vi "LVClass_CameraSet Get Parameter List.vi"(0 "CameraSet in":refnum<class "CameraSet.lvclass">, 11 "error in (no error)":errorcluster) -> (4 "CameraSet out":refnum<class "CameraSet.lvclass">, 8 "ListOfGettableParameter":T1[](array[typedef]), 15 "error out":errorcluster)   [LabVIEW 2020, in "CameraSet.lvclass"]
uses:
  CameraSet.lvclass
  CameraParametersSetup.ctl
  CameraParameters_Type.ctl
  CameraParameters.ctl
  CameraParameters_Authorization.ctl
  CameraParameters_OnFlyAuthorization.ctl
  CameraSet.lvclass/CameraSet.ctl
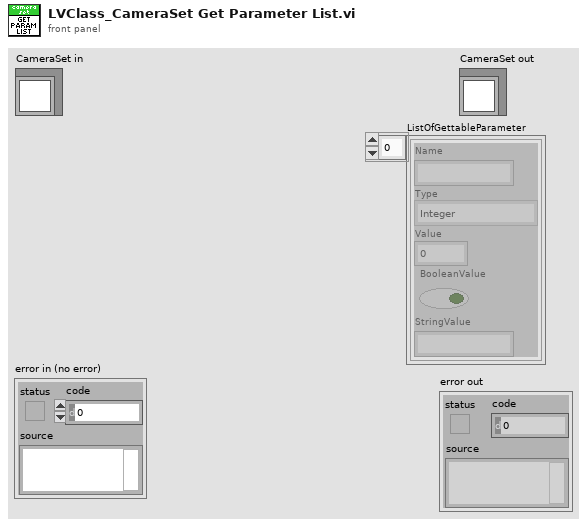
[diagram p1: front panel]
types:
  T1 = typedef "CameraParametersSetup.ctl" = cluster{"Name":string, "Type":T2, "Value":dbl, "BooleanValue":bool, "StringValue":string}
  T2 = typedef "CameraParameters_Type.ctl" = enum16{"Integer", "Real", "String", "Boolean"}
  T3 = typedef "CameraParameters_Authorization.ctl" = enum16{"Disable", "Gettable", "Settable - Gettable"}
  T4 = typedef "CameraParameters.ctl" = cluster{"Name":string, "Type":T2, "Authorization":T3, "OnFlyAuthorization":T5, "StringDefault":string, "Default":dbl, "Min":dbl, "Max":dbl, "Boolean":bool, "StringParameterList":string[]}
  T5 = typedef "CameraParameters_OnFlyAuthorization.ctl" = enum16{"None", "Gettable", "Settable", "Settable - Gettable"}
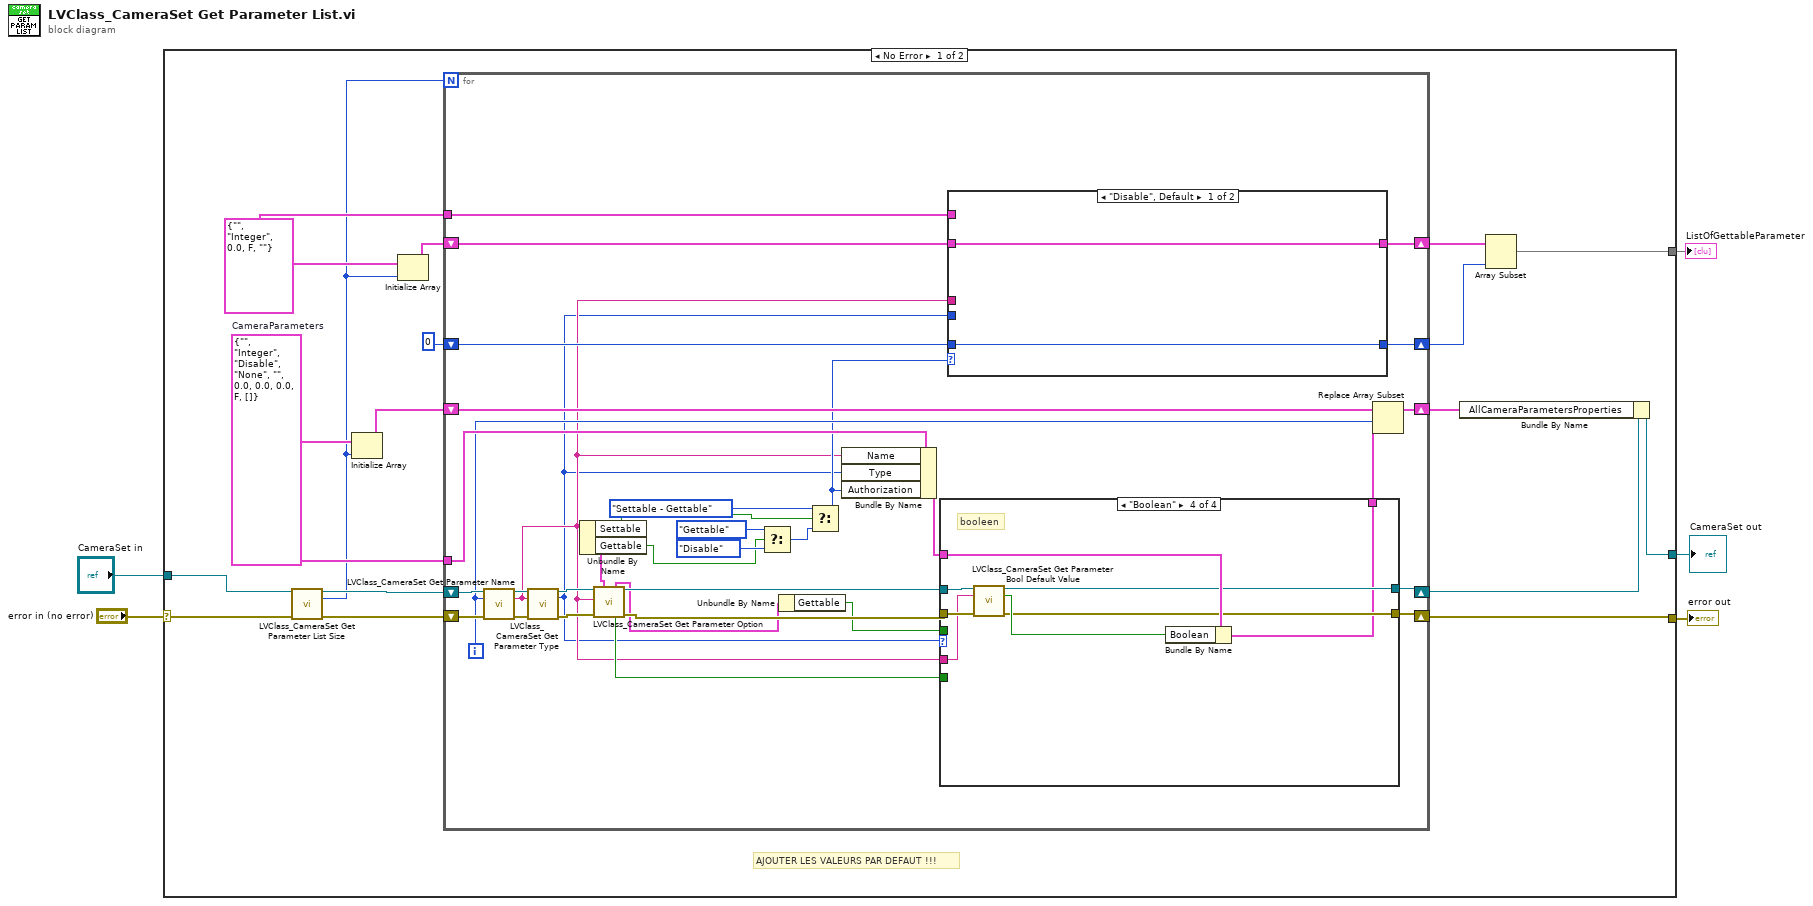
[diagram p0: block diagram]
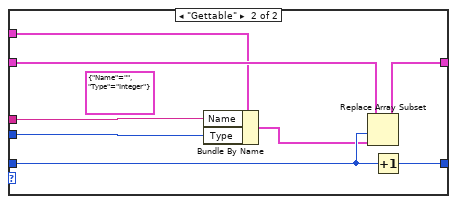
[diagram p2: hidden frame]
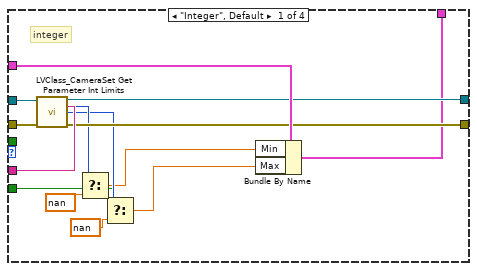
[diagram p3: hidden frame]
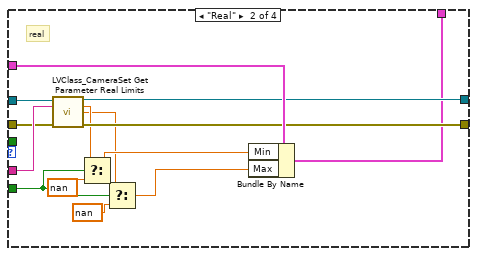
[diagram p4: hidden frame]
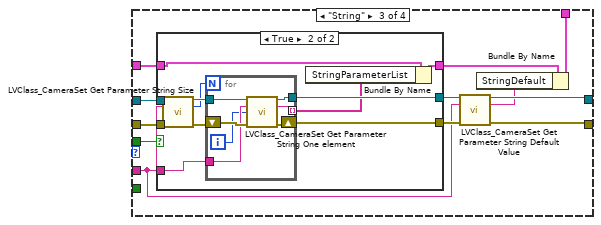
[diagram p5: hidden frame]
diagram:
  n1 = case shown="No Error" "error in (no error)" {
    selector: "error in (no error)" -> [w20 w137]
    tunnel: [w19 w137] -> w4
    tunnel: [w21 w136] -> w2
    tunnel: "CameraSet in" -> [w18 w136]
    tunnel: [w8 _] -> w1
    frame No Error {
      w7 = T1 {"Name"="", "Type"=enum."Integer", "Value"=0.0, "BooleanValue"=FALSE, "StringValue"=""} ("CameraParametersSetup")
      w14 = T4 {"Name"="", "Type"=enum."Integer", "Authorization"=enum."Disable", "OnFlyAuthorization"=enum."None", "StringDefault"="", "Default"=0.0, "Min"=0.0, "Max"=0.0, "Boolean"=FALSE, "StringParameterList"=[]}  # CameraParameters
      # "AJOUTER LES VALEURS PAR DEFAUT !!!"
      n2 = call "LVClass_CameraSet Get Parameter List Size.vi"("CameraSet.lvclass"=w18, "error in (no error)"=w20) -> ("CameraSet.lvclass"=w17:refnum<class "CameraSet.lvclass">, "size"=w6:i32, "error out"=w22:errorcluster)  [unwired: 11 in]
      n3 = Initialize Array(w14, w6) -> (w15:T4[])
      n4 = Initialize Array(w7, w6) -> (w10:T1[])
      n5 = for {
        N: w6 -> [_]
        tunnel: w14 -> [w52]
        shift-right: [w51] -> w19
        shift-left: w22 -> [w55]
        shift-right: [w50] -> w16
        shift-left: w17 -> [w56]
        shift-right: [w39] -> w13
        shift-left: w15 -> [w40]
        shift-right: [w35] -> w9
        shift-left: 0 -> [w36]
        shift-right: [w34] -> w11
        shift-left: w10 -> [w30]
        tunnel: w7 -> [w29]
        i -> [w37]
        n6 = call "LVClass_CameraSet Get Parameter Name.vi"("CameraSet.lvclass"=w56, "index"=w37, "error in (no error)"=w55) -> ("CameraSet.lvclass"=w54:refnum<class "CameraSet.lvclass">, "parameter_name"=w32:string, "error out"=w53:errorcluster)  [unwired: 10 in]
        n7 = call "LVClass_CameraSet Get Parameter Type.vi"("CameraSet.lvclass"=w54, "parameter_name"=w32, "error in (no error)"=w53) -> ("CameraSet.lvclass"=w49:refnum<class "CameraSet.lvclass">, "Type"=w31:T2, "error out"=w48:errorcluster)  [unwired: 10 in]
        n8 = call "LVClass_CameraSet Get Parameter Option.vi"("CameraSet.lvclass"=w49, "parameter_name"=w32, "error in (no error)"=w48) -> ("Settable-Gettable?"=w28:cluster{"Settable":bool, "Gettable":bool}, "Settable-Gettable on fly?"=w24:cluster{"Settable":bool, "Gettable":bool}, "CameraSet.lvclass"=w47:refnum<class "CameraSet.lvclass">, "minmax"=w41:bool, "error out"=w25:errorcluster)  [unwired: 6 in, 2 out]
        n9 = Unbundle By Name(w28) -> ("Settable"=w27:bool, "Gettable"=w26:bool)
        n10 = Select(t=CameraParameters_Authorization."Gettable" ("Authorization"), s=w26, f=CameraParameters_Authorization."Disable") -> (s? t:f=w44:T3)
        n11 = Unbundle By Name(w24) -> ("Gettable"=w23:bool)
        n12 = Select(t=CameraParameters_Authorization."Settable - Gettable", s=w27, f=w44) -> (s? t:f=w33:T3)
        n13 = Bundle By Name(cluster=w52, "Name"=w32, "Type"=w31, "Authorization"=w33) -> (w42:T4)
        n14 = case shown="\"Boolean\"" w31 {
          tunnel: w42 -> [w80 w94 w98 w134]
          tunnel: w32 -> [w79 w93 w100 w131]
          tunnel: [w78 w92 w102 w129] -> w51
          tunnel: w47 -> [w76 w90 w106 w133]
          tunnel: w25 -> [w75 w89 w105 w132]
          tunnel: [w77 w91 w103 w130] -> w50
          tunnel: w41 -> [w68 w82 _ _]
          tunnel: w23 -> [_ _ w96 _]
          tunnel: [w67 w81 w95 w128] -> w38
          frame "Integer", Default {
            # "integer"
            n15 = call "LVClass_CameraSet Get Parameter Int Limits.vi"("CameraSet.lvclass"=w76, "parameter_name"=w79, "error in (no error)"=w75) -> ("CameraSet.lvclass"=w77:refnum<class "CameraSet.lvclass">, "min"=w72:i32, "max"=w71:i32, "error out"=w78:errorcluster)  [unwired: 9 in]
            n16 = Select(t=w72, s=w68, f=nan) -> (s? t:f=w70:dbl)
            n17 = Select(t=w71, s=w68, f=nan) -> (s? t:f=w69:dbl)
            n18 = Bundle By Name(cluster=w80, "Min"=w70, "Max"=w69) -> (w67:T4)
          }
          frame "Real" {
            # "real"
            n19 = call "LVClass_CameraSet Get Parameter Real Limits.vi"("CameraSet.lvclass"=w90, "parameter_name"=w93, "error in (no error)"=w89) -> ("CameraSet.lvclass"=w91:refnum<class "CameraSet.lvclass">, "min"=w87:dbl, "max"=w85:dbl, "error out"=w92:errorcluster)  [unwired: 9 in]
            n20 = Select(t=w87, s=w82, f=nan) -> (s? t:f=w86:dbl)
            n21 = Select(t=w85, s=w82, f=nan) -> (s? t:f=w84:dbl)
            n22 = Bundle By Name(cluster=w94, "Min"=w86, "Max"=w84) -> (w81:T4)
          }
          frame "String" {
            n23 = case shown="True" w96 {
              tunnel: w106 -> [w109 w120]
              tunnel: w105 -> [w108 w119]
              tunnel: [w109 w115] -> w104
              tunnel: [w108 w114] -> w101
              tunnel: w100 -> [_ w113]
              tunnel: w98 -> [w107 w112]
              tunnel: [w107 w110] -> w97
              frame False {
              }
              frame True {
                n24 = call "LVClass_CameraSet Get Parameter String Size.vi"("CameraSet.lvclass"=w120, "parameter name"=w113, "error in (no error)"=w119) -> ("CameraSet.lvclass"=w118:refnum<class "CameraSet.lvclass">, "size"=w116:i32, "error out"=w117:errorcluster)  [unwired: 10 in]
                n25 = for {
                  N: w116 -> [_]
                  tunnel: w113 -> [w125]
                  tunnel: [w122] -> w115
                  tunnel: w118 -> [w127]
                  shift-right: [w121] -> w114
                  shift-left: w117 -> [w126]
                  tunnel: [w123] -> w111 mode=indexing
                  i -> [w124]
                  n26 = call "LVClass_CameraSet Get Parameter String One element.vi"("CameraSet.lvclass"=w127, "parameter name"=w125, "index"=w124, "error in (no error)"=w126) -> ("CameraSet.lvclass"=w122:refnum<class "CameraSet.lvclass">, "value"=w123:string, "error out"=w121:errorcluster)  [unwired: 9 in]
                }
                n27 = Bundle By Name(cluster=w112, "StringParameterList"=w111) -> (w110:T4)
              }
            }
            n28 = call "LVClass_CameraSet Get Parameter String Default Value.vi"("CameraSet.lvclass"=w104, "parameter name"=w100, "error in (no error)"=w101) -> ("CameraSet.lvclass"=w103:refnum<class "CameraSet.lvclass">, "Default value"=w99:string, "error out"=w102:errorcluster)  [unwired: 10 in]
            n29 = Bundle By Name(cluster=w97, "StringDefault"=w99) -> (w95:T4)
          }
          frame "Boolean" {
            # "booleen"
            n30 = call "LVClass_CameraSet Get Parameter Bool Default Value.vi"("CameraSet.lvclass"=w133, "parameter_name"=w131, "error in (no error)"=w132) -> ("CameraSet.lvclass"=w130:refnum<class "CameraSet.lvclass">, "Default value"=w135:bool, "error out"=w129:errorcluster)  [unwired: 10 in]
            n31 = Bundle By Name(cluster=w134, "Boolean"=w135) -> (w128:T4)
          }
        }
        n32 = case shown="\"Disable\", Default" w33 {
          tunnel: w36 -> [w57 w66]
          tunnel: [w57 w65] -> w35
          tunnel: [w58 w64] -> w34
          tunnel: w32 -> [_ w63]
          tunnel: w31 -> [_ w62]
          tunnel: w30 -> [w58 w60]
          tunnel: w29 -> [_ w59]
          frame "Disable", Default {
          }
          frame "Gettable" {
            (unwired) cluster{"Name":string, "Type":T2} {"Name"="", "Type"=enum."Integer"}
            n33 = Bundle By Name(cluster=w59, "Name"=w63, "Type"=w62) -> (w61:T1)
            n34 = Replace Array Subset(array=w60, new element=w61, index=w66) -> (w64:T1[])
            n35 = Increment(x=w66) -> (x+1=w65:i32)
          }
        }
        n36 = Replace Array Subset(array=w40, new element=w38, index=w37) -> (w39:T4[])
      }
      n37 = Bundle By Name(cluster=w16, "AllCameraParametersProperties"=w13) -> (w21:refnum<class "CameraSet.lvclass">)
      n38 = Array Subset(array=w11, length=w9) -> (w8:T1[])  [unwired: 1 in]
    }
    frame Error {
    }
  }
  "error out" <- w4
  "CameraSet out" <- w2
  "ListOfGettableParameter" <- w1
